vi "Panel.vi"(11 "IntegerPanel in":refnum<class "IntegerPanel.lvclass">) -> ()   [LabVIEW 2020, in "Conditum-Tools.lvlib" / "IntegerPanel.lvclass"]
uses:
  IntegerPanel.lvclass
  C:/dev/lv20CE/lv-conditum-tools/Conditum-Tools/ColumnPanel/ColumnPanel.lvclass
  C:/Program Files (x86)/National Instruments/LabVIEW 2020/vi.lib/IlluminatedG/IG OOPanel/OOPanel/Panel/Panel.lvclass
  ColumnPanel/Common Items.ctl
  <vilib>/IlluminatedG/IG OOPanel/OOPanel/Panel/Basic UI State.ctl
  IntegerPanel.lvclass/IntegerPanel.ctl
  Conditum-Clone/Columns/Type/Type.lvclass/Type.ctl
  Conditum-Clone/Columns/Integer/Integer Definition.ctl
  Conditum-Clone/Columns/Type/Definition.ctl
  Conditum-Clone/Attributes.ctl
  Conditum-Clone/Columns/Integer/Definition.ctl
  6db9cc57-236e-4a1f-9d91-1abc15db7500.vi
  Conditum-Clone/Columns/Integer/Integer.lvclass
  C:/dev/lv20CE/lv-conditum-tools/Conditum-Clone/Columns/Type/Type.lvclass
  Conditum-Clone/Columns/Type/Type.lvclass
  <vilib>/IlluminatedG/IG OOPanel/OOPanel/Panel/Panel.lvclass
  ColumnPanel/ColumnPanel.lvclass
  Conditum-Clone/Conditu2.lvlib
  <vilib>/IlluminatedG/IG OOPanel/OOPanel/OOPanel.lvlib
  C:/Program Files (x86)/National Instruments/LabVIEW 2020/vi.lib/IlluminatedG/IG OOPanel/OOPanel/ArrayPanel/ArrayPanel.lvclass
  C:/dev/lv20CE/lv-conditum-tools/Conditum-Tools/IntegerPanel/IntegerPanel.lvclass
panel:
  in  "Default Value":i64
  in  "Common Items":T1
  # "Integer"
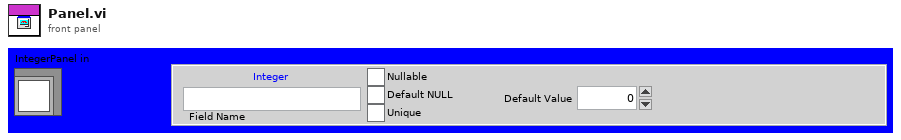
[diagram p1: front panel]
types:
  T1 = typedef "Conditum-Tools.lvlib/ColumnPanel.lvclass/Common Items.ctl" = cluster{"Name":string, "Nullable":bool, "Default NULL":bool, "Unique":bool}
  T2 = typedef "OOPanel.lvlib/Panel.lvclass/Basic UI State.ctl" = enum16{"Init", "Run", "Close"}
  T3 = typedef "Conditu2.lvlib/Columns.lvlib/Integer.lvclass/Integer Definition.ctl" = cluster{"Type":T4, "Attributes":T5, "Integer":T6}
  T4 = typedef "Conditu2.lvlib/Columns.lvlib/Type.lvclass/Definition.ctl" = cluster{"Name":string, "Nullable":bool, "Default NULL":bool}
  T5 = typedef "Conditu2.lvlib/Attributes.ctl" = cluster{"Primary Key":bool, "Unique":bool, "Foreign Key":bool, "Auto Increment":bool}
  T6 = typedef "Conditu2.lvlib/Columns.lvlib/Integer.lvclass/Definition.ctl" = cluster{"Default":i64}
  T7 = typedef "OOPanel.lvlib/Panel.lvclass/Panel Events.ctl" = cluster{"Visbility":refnum<user-event>, "Close":refnum<user-event>}
  T8 = typedef "Conditum-Tools.lvlib/ColumnPanel.lvclass/Events.ctl" = cluster{"Update":refnum<user-event>, "Value":refnum<user-event>, "Valid":refnum<user-event>, "Highlight":refnum<user-event>}
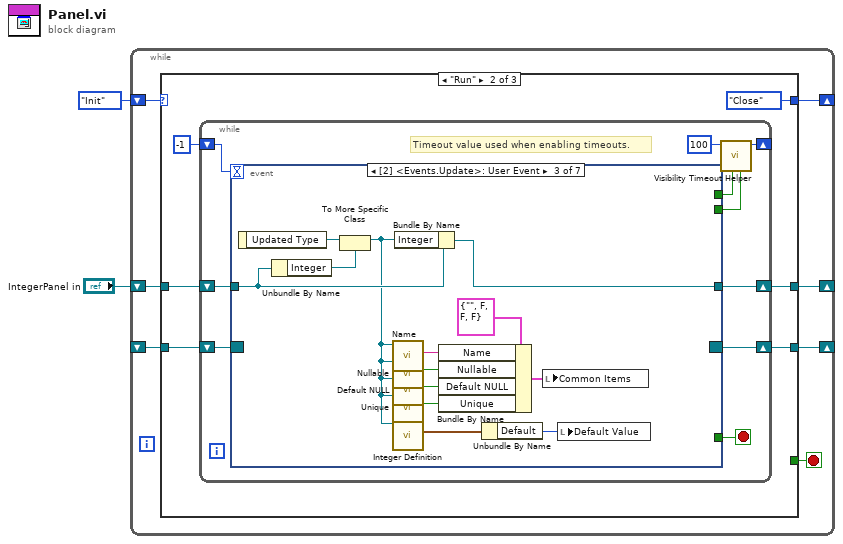
[diagram p0: block diagram]
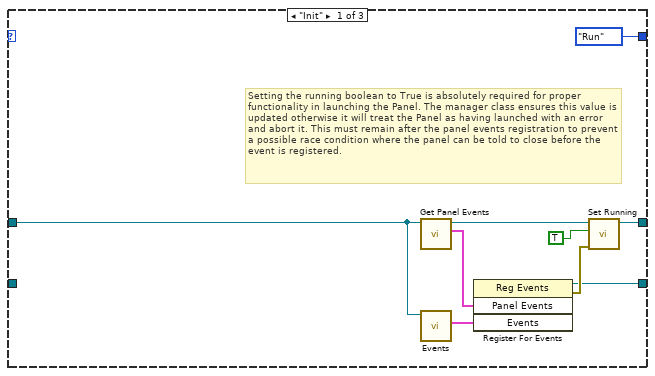
[diagram p2: hidden frame]
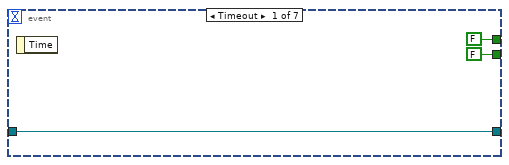
[diagram p3: hidden frame]
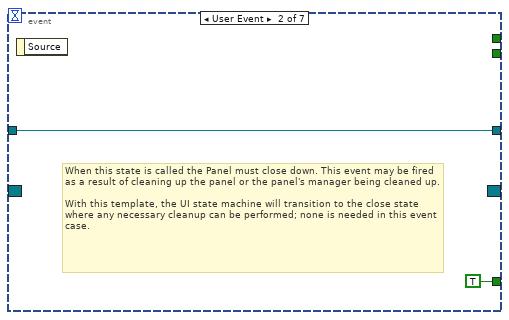
[diagram p4: hidden frame]
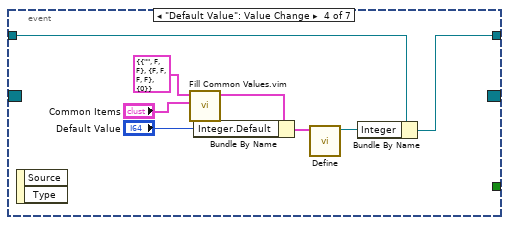
[diagram p5: hidden frame]
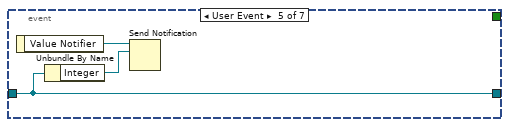
[diagram p6: hidden frame]
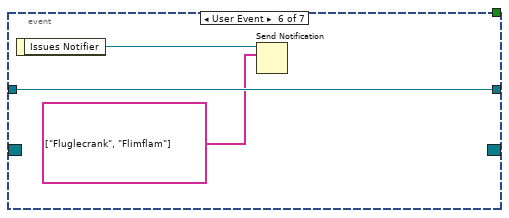
[diagram p7: hidden frame]
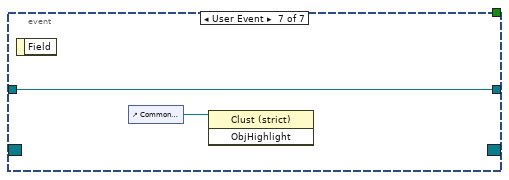
[diagram p8: hidden frame]
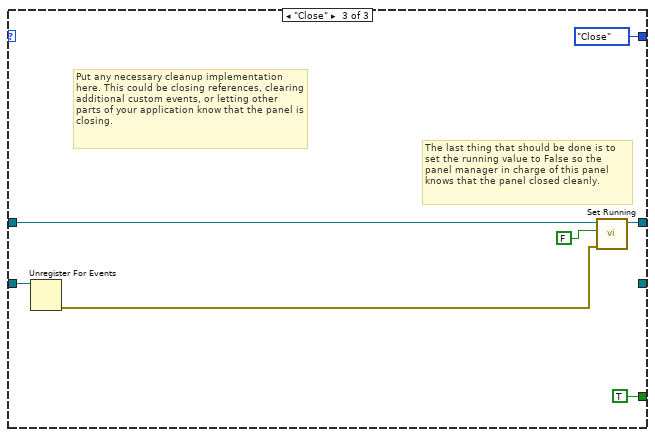
[diagram p9: hidden frame]
diagram:
  n1 = while {
    shift-right: [w8] -> _
    shift-left: _ -> [w9]
    shift-right: [w6] -> _
    shift-left: Basic_UI_State."Init" ("Basic UI State") -> [w7]
    shift-right: [w4] -> _
    shift-left: "IntegerPanel in" -> [w3]
    stop <- w5 stop-if-true
    n2 = case shown="\"Run\"" w7 {
      tunnel: w9 -> [_ w24 w71]
      tunnel: [w15 w22 _] -> w8
      tunnel: [Basic_UI_State."Run" ("Basic UI State") Basic_UI_State."Close" ("Basic UI State") Basic_UI_State."Close" ("Basic UI State")] -> w6
      tunnel: [_ _ TRUE] -> w5
      tunnel: [w14 w19 w69] -> w4
      tunnel: w3 -> [w10 w20 w70]
      frame "Init" {
        # "Setting the running boolean to True is absolutely required for proper functionality in launching the Panel. The manager class ensures this value is updated otherwise it will treat the Panel as having launched with an error and abort it. This must remain after the panel events registration to prevent a possible race condition where the panel can be told to close before the event is registered."
        n3 = call <vilib>:"Get Panel Events.vi"("Panel in"=w10) -> ("Panel Events"=w12:T7, "Panel out"=w13:refnum<class "IntegerPanel.lvclass">)  [unwired: 8 in, 1 out]
        n4 = call "Events.vi"("ColumnPanel in"=w10) -> ("Events"=w11:T8)  [unwired: 10 in]
        n5 = register-events(w12, w11) -> (reference out=w15:refnum<event-registration>, error out=w17:errorcluster)  [unwired: 2 in]
        n6 = call <vilib>:"Set Running.vi"("error in (no error)"=w17, "Running"=TRUE, "Panel in"=w13) -> ("Panel out"=w14:refnum<class "IntegerPanel.lvclass">)  [unwired: 7 in, 1 out]
      }
      frame "Run" {
        n7 = while {
          shift-right: [w30] -> w22
          shift-left: w24 -> [w31]
          shift-right: [w33] -> _
          shift-left: -1 ("Timeout") -> [w32]
          shift-right: [w25] -> w19
          shift-left: w20 -> [w26]
          stop <- w27 stop-if-true
          # "Timeout value used when enabling timeouts."
          n8 = event shown="[2] <Events.Update>: User Event" {
            selector: w31 -> [_ _ _ _ _ _ _]
            dyn-events: [_ _ _ _ _ _ _] -> w30
            timeout: w32 -> [_ _ _ _ _ _ _]
            tunnel: [FALSE _ _ _ _ _ _] -> w29
            tunnel: [FALSE _ _ _ _ _ _] -> w28
            tunnel: [_ TRUE _ _ _ _ _] -> w27
            tunnel: w26 -> [w35 w38 w50 w57 w63 w66 w68]
            tunnel: [w35 w38 w51 w58 w63 w66 w68] -> w25
            event Timeout {
              n9 = event-data() -> ()  [unwired: 1 in, 1 out]
            }
            event User Event {
              # "When this state is called the Panel must close down. This event may be fired as a result of cleaning up the panel or the panel's manager being cleaned up.\n\nWith this template, the UI state machine will transition to the close state where any necessary cleanup can be performed; none is needed in this event case."
              n10 = event-data() -> ()  [unwired: 1 in, 1 out]
            }
            event User Event {
              n11 = event-data() -> ("Updated Type"=w52:refnum<class "Type.lvclass">)  [unwired: 1 in]
              n12 = Unbundle By Name(w50) -> ("Integer"=w49:refnum<class "Integer.lvclass">)
              n13 = To More Specific Class(target class=w49, reference=w52) -> (specific class reference=w41:refnum<class "Integer.lvclass">)  [unwired: 1 in, 1 out]
              n14 = call "Name.vi"("Type in"=w41) -> ("Table Name"=w46:string)  [unwired: 10 in]
              n15 = call "Nullable.vi"("Type in"=w41) -> ("Nullable"=w45:bool)  [unwired: 10 in]
              n16 = call "Default NULL.vi"("Type in"=w41) -> ("Default NULL"=w44:bool)  [unwired: 10 in]
              n17 = call "Unique.vi"("Type in"=w41) -> ("Unique"=w43:bool)  [unwired: 10 in]
              n18 = call "Integer Definition.vi"("Integer in"=w41) -> ("Definition"=w42:T6)  [unwired: 10 in]
              n19 = Bundle By Name(cluster=w50, "Integer"=w41) -> (w51:refnum<class "IntegerPanel.lvclass">)
              n20 = Bundle By Name(cluster=T1 {"Name"="", "Nullable"=FALSE, "Default NULL"=FALSE, "Unique"=FALSE} ("Common Items"), "Name"=w46, "Nullable"=w45, "Default NULL"=w44, "Unique"=w43) -> (w47:T1)
              n21 = Unbundle By Name(w42) -> ("Default"=w40:i64)
              n22 = local write "Common Items"(w47) -> ()
              n23 = local write "Default Value"(w40) -> ()
            }
            event "Default Value": Value Change {
              n24 = event-data() -> ()  [unwired: 1 in, 2 out]
              n25 = call "Fill Common Values.vim"("Common Items"="Common Items", "Init Data Type"=T3 {"Type"={"Name"="", "Nullable"=FALSE, "Default NULL"=FALSE}, "Attributes"={"Primary Key"=FALSE, "Unique"=FALSE, "Foreign Key"=FALSE, "Auto Increment"=FALSE}, "Integer"={"Default"=0}} ("Init Data")) -> ("Init Data"=w55:T3)  [unwired: 9 in]
              n26 = Bundle By Name(cluster=w55, "Integer.Default"="Default Value") -> (w60:T3)
              n27 = call "Define.vi"("Integer Definition"=w60) -> ("Integer out"=w59:refnum<class "Integer.lvclass">)  [unwired: 10 in]
              n28 = Bundle By Name(cluster=w57, "Integer"=w59) -> (w58:refnum<class "IntegerPanel.lvclass">)
            }
            event User Event {
              n29 = event-data() -> ("Value Notifier"=w62:refnum<notifier>)  [unwired: 1 in]
              n30 = Unbundle By Name(w63) -> ("Integer"=w61:refnum<class "Integer.lvclass">)
              n31 = Send Notification(notification=w61, notifier=w62) -> ()  [unwired: 1 in, 2 out]
            }
            event User Event {
              n32 = event-data() -> ("Issues Notifier"=w65:refnum<notifier>)  [unwired: 1 in]
              n33 = Send Notification(notification=string[] ["Fluglecrank", "Flimflam"], notifier=w65) -> ()  [unwired: 1 in, 2 out]
            }
            event User Event {
              n34 = event-data() -> ()  [unwired: 1 in, 1 out]
              n35 = control-ref of="Common Items"() -> (w67:refnum<vi>)
              n36 = invoke class="Clust (strict)" method="ObjHighlight"(reference=w67) -> ()  [unwired: 2 in, 3 out]
            }
          }
          n37 = call <vilib>:"Visibility Timeout Helper.vi"("Update?"=w28, "Use Timeout?"=w29, "Visible Timeout mS"=100) -> ("Timeout"=w33:i32)  [unwired: 8 in]
        }
      }
      frame "Close" {
        # "Put any necessary cleanup implementation here. This could be closing references, clearing additional custom events, or letting other parts of your application know that the panel is closing."
        # "The last thing that should be done is to set the running value to False so the panel manager in charge of this panel knows that the panel closed cleanly."
        n38 = Unregister For Events(event registration refnum=w71) -> (error out=w73:errorcluster)  [unwired: 1 in]
        n39 = call <vilib>:"Set Running.vi"("error in (no error)"=w73, "Running"=FALSE, "Panel in"=w70) -> ("Panel out"=w69:refnum<class "IntegerPanel.lvclass">)  [unwired: 7 in, 1 out]
      }
    }
  }
